vi "Read Data.vi"(0 "UART Driver in":refnum<class "UART Driver.lvclass">, 1 "Port Number":u8=1, 5 "Rx byte count":u32, 11 "error in":errorcluster) -> (4 "UART Driver out":refnum<class "UART Driver.lvclass">, 6 "Receive Data":string, 15 "error out":errorcluster)   [LabVIEW 2012, in "UART_Host_Driver.lvlib" / "UART Driver.lvclass"]
doc: "Reads the specified number of bytes from the device or interface specified by the Channel Number and returns the data in read buffer.\n\nMust call UART Initialize.vi, UART Configure Port.vi, and UART Read Data.vi prior to calling UART Read Data.vi.\n\nNote: Port Number 255 means to transmit to all of the ports configured in the UART Initialize.vi."
uses:
  UART Driver.lvclass
  Typedefs/FPGA VI Reference.ctl
  UART Driver.lvclass/UART Driver.ctl
  <vilib>/Utility/error.llb/Error Cluster From Error Code.vi
  <vilib>/rvi/errors/niLvFpgaAdjustHostInterfaceError.vi
  <vilib>/rvi/interface/nirviMethod/nirviMethod.xnode
  <vilib>/ErrorRing/Error Ring.xnode
  UART_Host_Driver.lvlib
  <vilib>/FPGAPlugInAG/Dynamic/niLvFpga_ReadFifo_Dynamic.vi
  <vilib>/rvi/errors/niLvFpgaMergeErrorWithErrorCode.vi
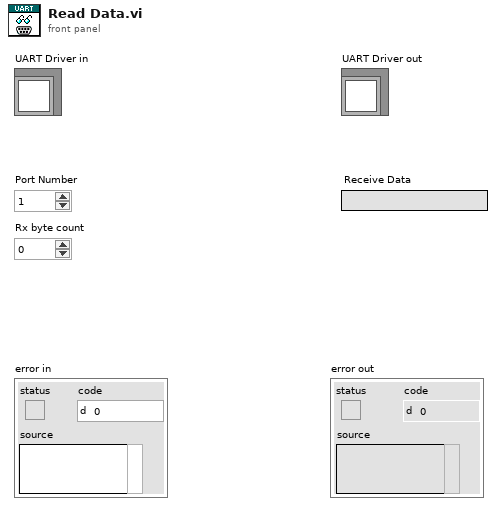
[diagram p1: front panel]
types:
  T1 = typedef "UART_Host_Driver.lvlib/FPGA VI Reference.ctl" = refnum<k20>
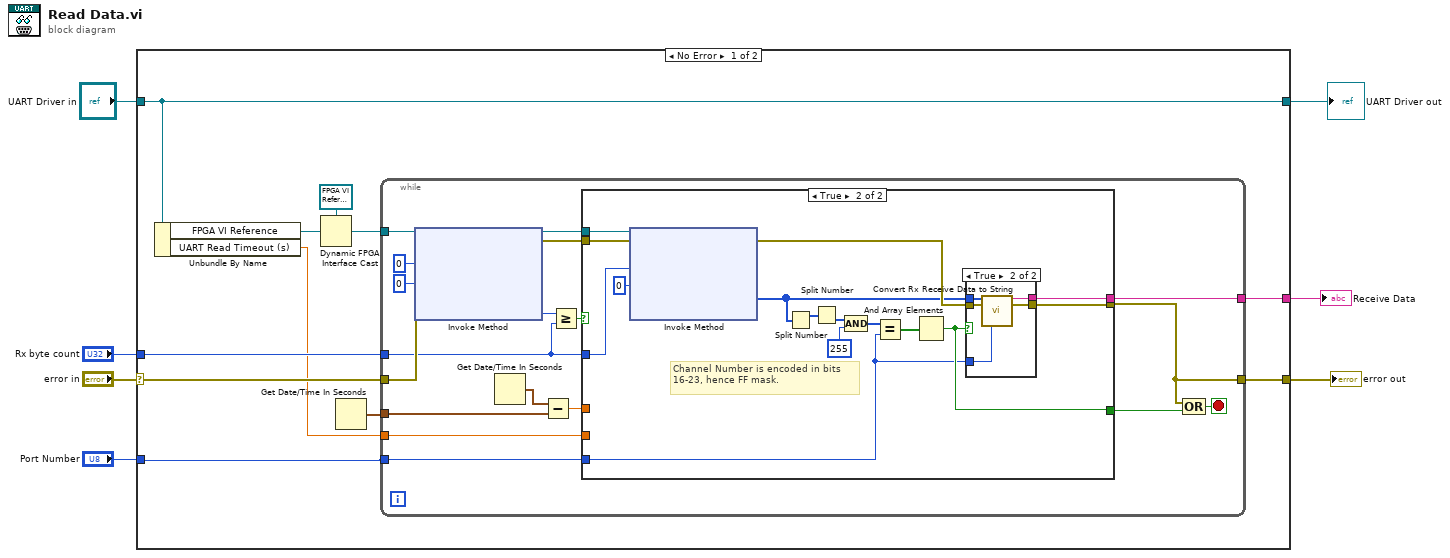
[diagram p0: block diagram]
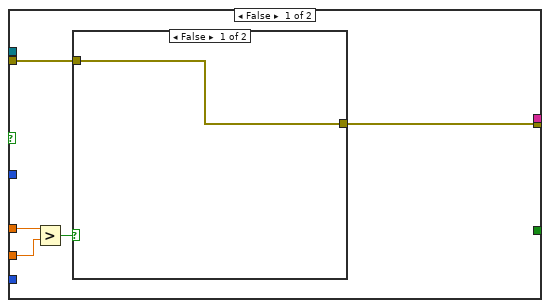
[diagram p2: hidden frame]
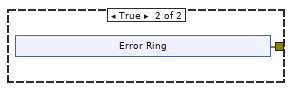
[diagram p3: hidden frame]
diagram:
  n1 = case shown="No Error" "error in" {
    selector: "error in" -> [w14 w70]
    tunnel: [w13 w70] -> w6
    tunnel: [w18 w69] -> w4
    tunnel: "UART Driver in" -> [w18 w69]
    tunnel: "Rx byte count" -> [w11 _]
    tunnel: [w12 _] -> w3
    tunnel: "Port Number" -> [w9 _]
    frame No Error {
      n2 = Unbundle By Name(w18) -> ("FPGA VI Reference"=w17:refnum<k20>, "UART Read Timeout (s)"=w10:dbl)
      n3 = Dynamic FPGA Interface Cast(Session In=T1 refnum ("FPGA VI Reference"), Type=w17) -> (Session Out=w15:T1)
      n4 = Get Date/Time In Seconds() -> (seconds since 1Jan1904=w8:timestamp)
      n5 = while {
        tunnel: w15 -> [w36]
        tunnel: w14 -> [w35]
        tunnel: w11 -> [w29]
        tunnel: [w20] -> w13
        tunnel: w10 -> [w23]
        tunnel: w8 -> [w26]
        tunnel: w9 -> [w21]
        tunnel: [w19] -> w12
        stop <- w22 stop-if-true
        n6 = xnode "Invoke Method"("FPGA VI Reference In"=w36, "error in"=w35, "Number of Elements"=u32 0, "Timeout (ms)"=0) -> ("FPGA VI Reference Out"=w32:T1, "error out"=w28:errorcluster, "Elements Remaining"=w31:u32)  [unwired: 1 out]
        n7 = Get Date/Time In Seconds() -> (seconds since 1Jan1904=w25:timestamp)
        n8 = Subtract(x=w25, y=w26) -> (x-y=w24:dbl)
        n9 = Greater Or Equal?(x=w31, y=w29) -> (x >= y?=w30:bool)
        n10 = case shown="True" w30 {
          tunnel: w32 -> [_ w62]
          tunnel: w29 -> [_ w61]
          tunnel: w28 -> [w38 w59]
          tunnel: [w37 w52] -> w20
          tunnel: [_ w50] -> w27
          tunnel: w24 -> [w41 _]
          tunnel: w23 -> [w40 _]
          tunnel: w21 -> [_ w48]
          tunnel: [_ w49] -> w19
          frame False {
            n11 = Greater?(x=w41, y=w40) -> (0:w39:bool)
            n12 = case shown="False" w39 {
              tunnel: w38 -> [w42 _]
              tunnel: [w42 w43] -> w37
              frame False {
              }
              frame True {
                n13 = xnode "Error Ring"() -> ("error out"=w43:errorcluster)
              }
            }
          }
          frame True {
            # "Channel Number is encoded in bits 16-23, hence FF mask."
            n14 = xnode "Invoke Method"("FPGA VI Reference In"=w62, "error in"=w59, "Number of Elements"=w61, "Timeout (ms)"=0) -> ("error out"=w54:errorcluster, "Data"=w53:u32[])  [unwired: 2 out]
            n15 = Split Number(x=w53) -> (hi(x)=w56:u16[])  [unwired: 1 out]
            n16 = Split Number(x=w56) -> (lo(x)=w55:u8[])  [unwired: 1 out]
            n17 = Compound Arithmetic op=AND(w55, u8 255 ("Numeric")) -> (w57:u8[])
            n18 = Equal?(x=w57, y=w48) -> (x = y?=w51:bool[])
            n19 = And Array Elements(Boolean array=w51) -> (logical AND=w50:bool)
            n20 = case shown="True" w50 {
              tunnel: w54 -> [w63 w68]
              tunnel: w53 -> [_ w67]
              tunnel: [_ w66] -> w49
              tunnel: [w63 w65] -> w52
              tunnel: w48 -> [_ w64]
              frame False {
              }
              frame True {
                n21 = call "Convert Rx Receive Data to String.vi"("Rx_Data"=w67, "Port Number"=w64, "error in"=w68) -> ("String"=w66:string, "error out"=w65:errorcluster)  [unwired: 11 in]
              }
            }
          }
        }
        n22 = Compound Arithmetic op=OR(w20, w27) -> (w22:bool)
      }
    }
    frame Error {
    }
  }
  "error out" <- w6
  "UART Driver out" <- w4
  "Receive Data" <- w3
